vi "6-1 Mux.vi"(0 "input 0":bool, 1 "input 1":bool, 2 "input 2":bool, 3 "input 3":bool, 4 "input 4":bool, 5 "input 5":bool, 6 "select":u8) -> (14 "output":bool)   [LabVIEW 2015]
doc: "Sets the <B>output</B> to the <B>input</B> that you specify in the <B>select</B> parameter."
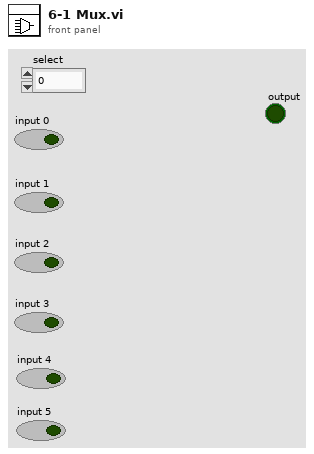
[diagram p1: front panel]
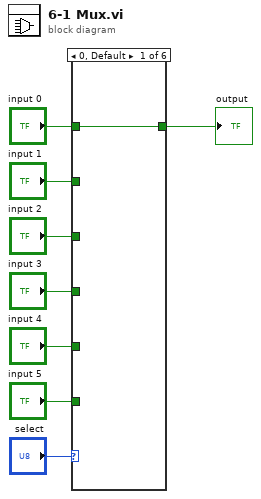
[diagram p0: block diagram]
diagram:
  n1 = case shown="0, Default" "select" {
    tunnel: "input 0" -> [w9 _ _ _ _ _]
    tunnel: "input 1" -> [_ w10 _ _ _ _]
    tunnel: "input 2" -> [_ _ w11 _ _ _]
    tunnel: "input 3" -> [_ _ _ w12 _ _]
    tunnel: [w9 w10 w11 w12 w13 w14] -> w4
    tunnel: "input 4" -> [_ _ _ _ w13 _]
    tunnel: "input 5" -> [_ _ _ _ _ w14]
    frame 0, Default {
    }
    frame 1 {
    }
    frame 2 {
    }
    frame 3 {
    }
    frame 4 {
    }
    frame 5 {
    }
  }
  "output" <- w4
